vi "Einheit an Kanal anpassen.vi"(8 "Indizes":i32[](array[numeric]), 9 "Einheit":string, 10 "Konzentration IST":dbl, 11 "Aktuelle Gasliste gesamt":T1[](array[typedef])) -> (3 "Konzentrationen":dbl[](array[numeric]))   [LabVIEW 2020, in "System Einstellungen V2.lvlib"]
uses:
  System Einstellungen V2.lvlib
  Visualisierungs Elemente/String - Ausgabefeld.ctl
  <vilib>/regexp/Match Regular Expression.xnode
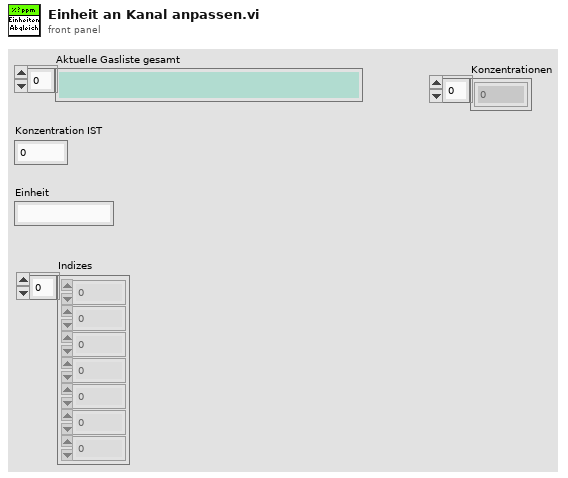
[diagram p1: front panel]
types:
  T1 = typedef "String - Ausgabefeld.ctl" = string
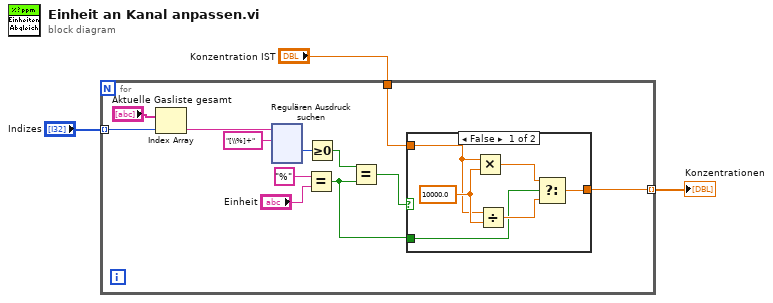
[diagram p0: block diagram]
diagram:
  n1 = for {
    tunnel: "Indizes" -> [w9] mode=indexing
    tunnel: "Konzentration IST" -> [w7]
    tunnel: [w4] -> w1 mode=indexing
    n2 = Index Array(array="Aktuelle Gasliste gesamt", index=w9) -> (element=w12:T1)
    n3 = xnode "Regulären Ausdruck suchen"("Eingangs-String"=w12, "Regulärer Ausdruck"="[\\%]+") -> ("Offset nach Übereinstimmung"=w15:i32)  [unwired: 4 in, 4 out]
    n4 = Equal?(x="%", y="Einheit") -> (x = y?=w6:bool)
    n5 = Greater Or Equal To 0?(x=w15) -> (x >= 0?=w5:bool)
    n6 = Equal?(x=w5, y=w6) -> (x = y?=w8:bool)
    n7 = case shown="False" w8 {
      tunnel: w7 -> [w19 w22]
      tunnel: [w17 w22] -> w4
      tunnel: w6 -> [w16 _]
      frame False {
        w20 = 10000.0 ("t")
        n8 = Multiply(x=w19, y=w20) -> (x*y=w21:dbl)
        n9 = Divide(x=w19, y=w20) -> (x/y=w18:dbl)
        n10 = Select(t=w21, s=w16, f=w18) -> (s? t:f=w17:dbl)
      }
      frame True {
      }
    }
  }
  "Konzentrationen" <- w1
